vi "onceavo.vi"() -> ()   [LabVIEW 2012]
panel:
  out "XY Graph":cluster{"Y":dbl[], "Y":dbl[]}[](graph)
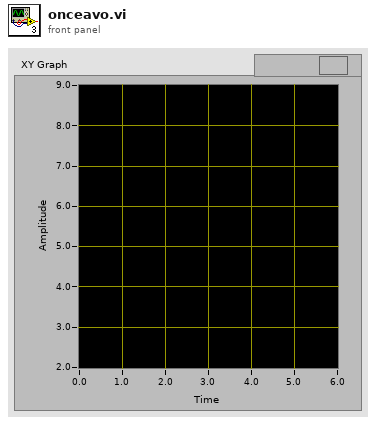
[diagram p1: front panel]
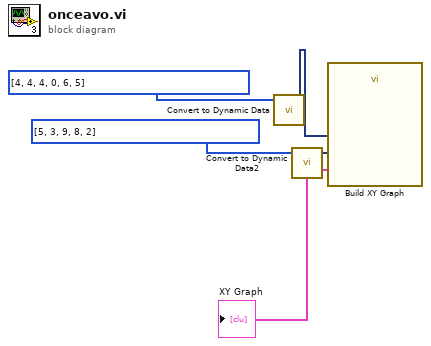
[diagram p0: block diagram]
diagram:
  n1 = call "Convert to Dynamic Data"("Array"=i32[] [4, 4, 4, 0, 6, 5]) -> ("Dynamic Data Type"=w4:dynamicdata)  [unwired: 3 in]
  n2 = call "Convert to Dynamic Data2"("Array"=i32[] [5, 3, 9, 8, 2]) -> ("Dynamic Data Type"=w2:dynamicdata)  [unwired: 3 in]
  n3 = call "Build XY Graph"("Y Input"=w2, "X Input"=w4) -> ("XY Graph"=→"XY Graph":cluster{"Y":dbl[], "Y":dbl[]}[])  [unwired: 3 in, 6 out]
